vi "HIOKI PW3390 Conf AutoRange type.vi"(0 "VISA Resource":refnum<visa-resource-name>, 1 "Set/Query (F: Set)":bool, 5 "AutoRange Type (1: Narrow)":enum16{"WIDE", "NARROW"}(ring)=enum."NARROW", 11 "error in (no error)":errorcluster, 12 "OPC query (T: ON)":bool=TRUE, 13 "Error Out (F: Off)":bool) -> (4 "VISA Resource out":refnum<visa-resource-name>, 6 "AutoRange Type out":enum16{"WIDE", "NARROW"}(ring)=enum."NARROW", 15 "error out":errorcluster)   [LabVIEW 2009]
doc: "Set/Query\n Set: Send the setting commands for the device.\n Query: Query the setting of the device.\n\nAutoRange Type\n Sets the AutoRange pattern."
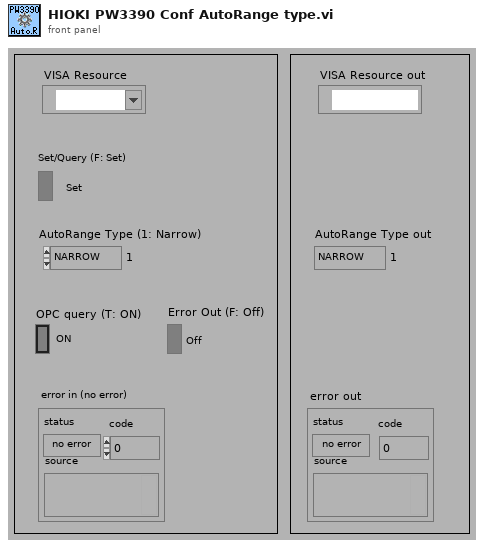
[diagram p1: front panel]
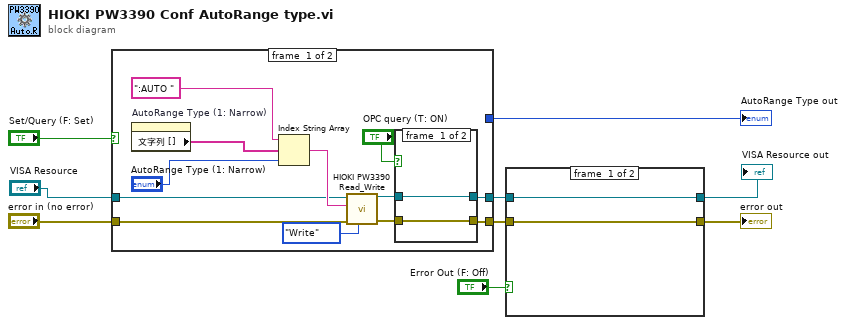
[diagram p0: block diagram]
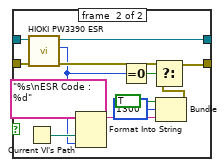
[diagram p2: hidden frame]
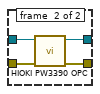
[diagram p3: hidden frame]
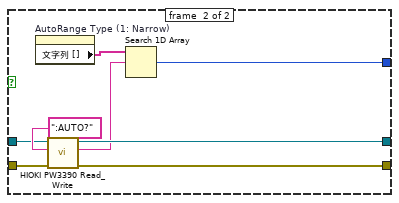
[diagram p4: hidden frame]
diagram:
  n1 = case shown="FALSE" "Set/Query (F: Set)" {
    tunnel: "error in (no error)" -> [w20 w32]
    tunnel: [w12 w34] -> w5
    tunnel: [w13 w33] -> w4
    tunnel: [_ w29] -> w7
    tunnel: "VISA Resource" -> [w15 w28]
    frame #0 {
      n2 = property on="AutoRange Type (1: Narrow)" class="Enum (strict)"() -> ("文字列 []"=w16:string[])  [unwired: 2 in, 2 out]
      n3 = Index String Array(1:"AutoRange Type (1: Narrow)", 2:w16, 3:":AUTO ") -> (0:w17:string)
      n4 = call <instrlib>:"HIOKI PW3390 Read_Write.vi"("Read/Write"=enum16{"Read", "Write"}."Write", "error in (no error)"=w20, "data in"=w17, "VISA Resource"=w15) -> ("error out"=w10:errorcluster, "VISA Resource out"=w11:refnum<visa-resource-name>)  [unwired: 5 in, 1 out]
      n5 = case shown="TRUE" "OPC query (T: ON)" {
        tunnel: [w23 w27] -> w13
        tunnel: [w22 w26] -> w12
        tunnel: w11 -> [w23 w25]
        tunnel: w10 -> [w22 w24]
        frame #0 {
        }
        frame #1 {
          n6 = call <instrlib>:"HIOKI PW3390 OPC.vi"("error in (no error)"=w24, "VISA Resource"=w25) -> ("error out"=w26:errorcluster, "VISA Resource out"=w27:refnum<visa-resource-name>)  [unwired: 7 in, 1 out]
        }
      }
    }
    frame #1 {
      n7 = property on="AutoRange Type (1: Narrow)" class="Enum (strict)"() -> ("文字列 []"=w31:string[])  [unwired: 2 in, 2 out]
      n8 = call <instrlib>:"HIOKI PW3390 Read_Write.vi"("error in (no error)"=w32, "data in"=":AUTO?", "VISA Resource"=w28) -> ("error out"=w34:errorcluster, "data out"=w30:string, "VISA Resource out"=w33:refnum<visa-resource-name>)  [unwired: 6 in]
      n9 = Search 1D Array(1D array=w31, element=w30) -> (index of element=w29:i32)  [unwired: 1 in]
    }
  }
  "AutoRange Type out" <- w7
  n10 = case shown="TRUE" "Error Out (F: Off)" {
    tunnel: w4 -> [w37 w50]
    tunnel: w5 -> [w36 w49]
    tunnel: [w36 w39] -> w3
    tunnel: [w37 w48] -> w2
    frame #0 {
    }
    frame #1 {
      n11 = Current VI's Path() -> (path=w46:path)
      n12 = call <instrlib>:"HIOKI PW3390 ESR.vi"("error in (no error)"=w49, "VISA Resource"=w50) -> ("error out"=w40:errorcluster, "Output Value"=w38:u8, "VISA Resource out"=w48:refnum<visa-resource-name>)  [unwired: 6 in, 1 out]
      n13 = Format Into String(format string="%s\nESR Code : %d", w46, w38) -> (resulting string=w42:string)  [unwired: 2 in, 1 out]
      n14 = Equal To 0?(x=w38) -> (x = 0?=w47:bool)
      n15 = Bundle("status"=TRUE, "code"=1300, w42) -> (w41:cluster{"status":bool, "code":i32, string})  [unwired: 1 in]
      n16 = Select(t=w40, s=w47, f=w41) -> (s? t:f=w39:errorcluster)
    }
  }
  "error out" <- w3
  "VISA Resource out" <- w2
